vi "Initialize.vi"(6 "Actor Name":string, 7 "Host Name":string, 8 "error in (no error)":errorcluster, 10 "Application Data":path, 11 "Message Broker":refnum<class "Message Broker Interface Ref.lvclass">) -> (0 "error out":errorcluster, 3 "Terminal Message out":refnum<class "Terminal Message.lvclass">)   [LabVIEW 2016, in "CLD Exam - ATM.lvlib" / "Terminal Message.lvclass"]
uses:
  Terminal Message.lvclass
  D:/Repos/Stream/software/Mediator/Classes/Mediated Actor/Mediated Actor.lvclass
  Mediator/Classes/Message Broker Interface Ref/Message Broker Interface Ref.lvclass
  D:/Repos/Stream/software/Mediator/Classes/Message Broker Interface/Message Broker Interface.lvclass
  Log/Application Log/Log Level.ctl
  Mediator/Classes/Message String/Message String.lvclass
  D:/Repos/Stream/software/Mediator/Classes/Message Interface/Message Interface.lvclass
  Terminal Message.lvclass/Terminal Message.ctl
  Mediator/Classes/Message Transport Queue/Message Transport Queue.lvclass
  D:/Repos/Stream/software/Mediator/Classes/Message Transport Interface/Message Transport Interface.lvclass
  Mediator/Classes/Mediated Actor/Mediated Actor.lvclass
  Log/Application Log/Application Log.lvclass
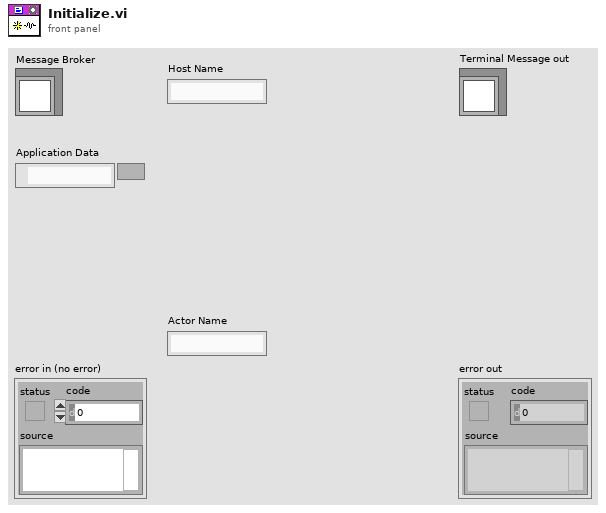
[diagram p1: front panel]
types:
  T1 = typedef "Stream Log.lvlib/Application Log.lvclass/Log Level.ctl" = enum16{"Imperative", "Major", "Minor", "Debug", "Off"}
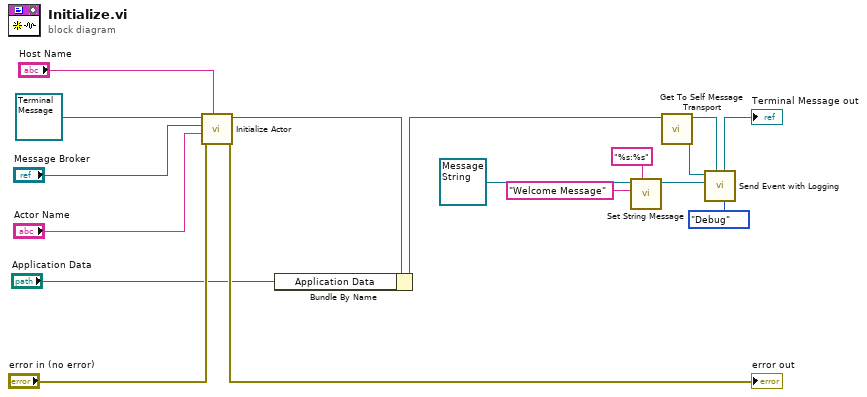
[diagram p0: block diagram]
diagram:
  n1 = call-dynamic "Initialize Actor.vi"("Host Name"="Host Name", "error in (no error)"="error in (no error)", "Actor Name"="Actor Name", "Message Broker Interface"="Message Broker", "Terminal Message in"=refnum<class "Terminal Message.lvclass"> refnum) -> ("error out"=→"error out":errorcluster, "Terminal Message out"=w10:refnum<class "Terminal Message.lvclass">)  [unwired: 5 in]
  n2 = Bundle By Name(cluster=w10, "Application Data"="Application Data") -> (w8:refnum<class "Terminal Message.lvclass">)
  n3 = call "Set String Message.vi"("Format"="%s:%s", "Name"="Welcome Message", "Message String in"=refnum<class "Message String.lvclass"> refnum ("Stream Mediator.lvlib:Message String.lvclass")) -> ("Message String out"=w4:refnum<class "Message String.lvclass">)  [unwired: 7 in, 1 out]
  n4 = call "Get To Self Message Transport.vi"("Mediated Actor in"=w8) -> ("To Self"=w5:refnum<class "Message Transport Queue.lvclass">, "Mediated Actor out"=w3:refnum<class "Terminal Message.lvclass">)  [unwired: 9 in]
  n5 = call "Send Event with Logging.vi"("Global Log Level"=Log_Level."Debug", "Mediated Actor in"=w3, "Message"=w4, "Message Transport Interface in"=w5) -> ("Mediated Actor out"=→"Terminal Message out":refnum<class "Terminal Message.lvclass">)  [unwired: 6 in, 1 out]
